vi "Temp_indicator.vi"() -> ()   [LabVIEW 2018]
uses:
  <vilib>/LabVIEW Interface for Arduino/Type Defs/Connection Type.ctl
  <vilib>/LabVIEW Interface for Arduino/Type Defs/Board Type.ctl
  <vilib>/LabVIEW Interface for Arduino/Type Defs/Pin Mode.ctl
  <vilib>/LabVIEW Interface for Arduino/LabVIEW Interface for Arduino.lvlib
panel:
  out "Temperature Gragh":dbl(graph)
  out "Temp":dbl(slide) scale=0.0..100.0
  out "Voltage":dbl(knob) scale=0.0..5.0
  in  "Max":dbl
  in  "Min":dbl
  out "Message":string
  out "Cold":bool
  out "Normal":bool
  out "Hot":bool
  out "Current Temperature":dbl
  in  "Analog":u8
  in  "Board Type (Uno)":T1
  in  "Connection Type (USB/Serial)":T2
  in  "VISA resource":refnum<visa-resource-name>
  in  "Baud Rate (115200)":u32=115200
  in  "stop":bool
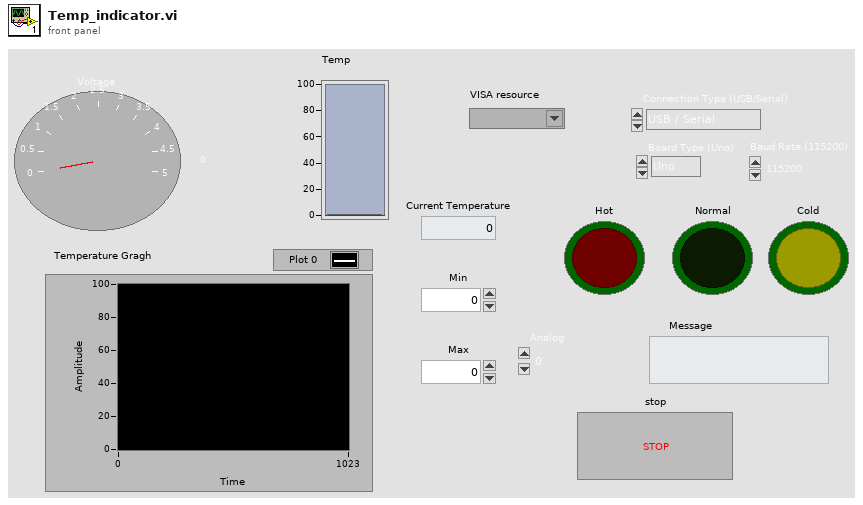
[diagram p1: front panel]
types:
  T1 = typedef "LabVIEW Interface for Arduino.lvlib/Board Type.ctl" = enum16{"Uno", "Dimuelanove w/Atmega 328", "Mega 2560"}
  T2 = typedef "LabVIEW Interface for Arduino.lvlib/Connection Type.ctl" = enum8{"USB / Serial", "XBEE", "BlueSmirf (Bluetooth)"}
  T3 = typedef "LabVIEW Interface for Arduino.lvlib/Pin Mode.ctl" = enum8{"Input", "Output"}
  T4 = typedef "LabVIEW Interface for Arduino.lvlib/Arduino Resource.ctl" = cluster{"VISA resource":refnum<visa-resource-name>, "Board Type":T1, "Connection Type":enum8{"USB / Serial"}, "Bytes Per Packet (15)":u8}
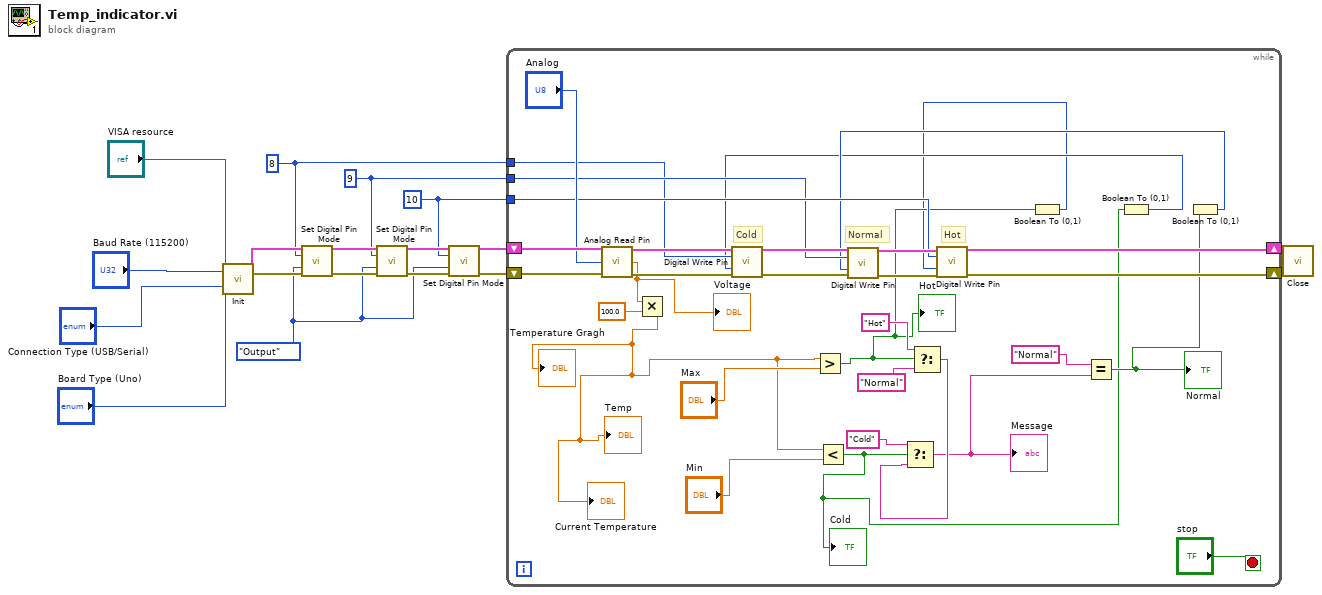
[diagram p0: block diagram]
diagram:
  w3 = u8 10 ("Digital I/O Pin")
  w2 = u8 9 ("Digital I/O Pin")
  w1 = u8 8 ("Digital I/O Pin")
  w4 = Pin_Mode."Output" ("Pin Mode (Input)")
  n1 = call <vilib>:"Init.vi"("VISA resource"="VISA resource", "Baud Rate (115200)"="Baud Rate (115200)", "Board Type (Uno)"="Board Type (Uno)", "Connection Type (USB/Serial)"="Connection Type (USB/Serial)") -> ("Arduino Resource"=w12:T4, "error out"=w11:errorcluster)  [unwired: 14 in]
  n2 = call <vilib>:"Set Digital Pin Mode.vi"("Arduino Resource"=w12, "Digital I/O Pin"=w1, "Pin Mode (Input)"=w4, "error in"=w11) -> ("Arduino Resource"=w18:T4, "error out"=w17:errorcluster)  [unwired: 10 in]
  n3 = call <vilib>:"Set Digital Pin Mode.vi"("Arduino Resource"=w18, "Digital I/O Pin"=w2, "Pin Mode (Input)"=w4, "error in"=w17) -> ("Arduino Resource"=w16:T4, "error out"=w15:errorcluster)  [unwired: 10 in]
  n4 = call <vilib>:"Set Digital Pin Mode.vi"("Arduino Resource"=w16, "Digital I/O Pin"=w3, "Pin Mode (Input)"=w4, "error in"=w15) -> ("Arduino Resource"=w14:T4, "error out"=w13:errorcluster)  [unwired: 10 in]
  n5 = while {
    shift-right: [w42] -> w10
    shift-left: w14 -> [w46]
    shift-right: [w41] -> w9
    shift-left: w13 -> [w45]
    tunnel: w3 -> [w38]
    tunnel: w2 -> [w37]
    tunnel: w1 -> [w36]
    stop <- "stop" stop-if-true
    # "Hot"
    # "Normal"
    # "Cold"
    n6 = call <vilib>:"Analog Read Pin.vi"("Arduino Resource"=w46, "Analog Input Pin (0)"="Analog", "error in"=w45) -> ("Arduino Resource"=w44:T4, "Voltage"=w19:dbl, "error out"=w43:errorcluster)  [unwired: 10 in]
    "Voltage" <- w19
    n7 = Multiply(x=w19, y=100.0) -> (x*y=w20:dbl)
    "Current Temperature" <- w20
    "Temp" <- w20
    "Temperature Gragh" <- w20
    n8 = Greater?(x=w20, y="Max") -> (0:w23:bool)
    "Hot" <- w23
    n9 = Less?(x=w20, y="Min") -> (x < y?=w25:bool)
    "Cold" <- w25
    n10 = Select(t="Hot", s=w23, f="Normal") -> (s? t:f=w30:string)
    n11 = Select(t="Cold", s=w25, f=w30) -> (s? t:f=w28:string)
    "Message" <- w28
    n12 = Boolean To (0,1)(Boolean=w23) -> (0, 1=w22:i16)
    n13 = Equal?(x="Normal", y=w28) -> (x = y?=w27:bool)
    "Normal" <- w27
    n14 = Boolean To (0,1)(Boolean=w25) -> (0, 1=w24:i16)
    n15 = call <vilib>:"Digital Write Pin.vi"("Arduino Resource"=w44, "Digital I/O Pin (0)"=w36, "Value (0)"=w24, "error in"=w43) -> ("Arduino Resource"=w50:T4, "error out"=w49:errorcluster)  [unwired: 10 in]
    n16 = Boolean To (0,1)(Boolean=w27) -> (0, 1=w26:i16)
    n17 = call <vilib>:"Digital Write Pin.vi"("Arduino Resource"=w50, "Digital I/O Pin (0)"=w37, "Value (0)"=w26, "error in"=w49) -> ("Arduino Resource"=w48:T4, "error out"=w47:errorcluster)  [unwired: 10 in]
    n18 = call <vilib>:"Digital Write Pin.vi"("Arduino Resource"=w48, "Digital I/O Pin (0)"=w38, "Value (0)"=w22, "error in"=w47) -> ("Arduino Resource"=w42:T4, "error out"=w41:errorcluster)  [unwired: 10 in]
  }
  n19 = call <vilib>:"Close.vi"("Arduino Resource"=w10, "error in"=w9) -> ()  [unwired: 13 in, 1 out]
